vi "CRYRta weights interpolate.vi"(9 "Weights in dB":dbl[](array[numeric]) format="%.2f", 10 "Frequencies of weights array":dbl[](array[numeric]) format="%.2f", 11 "Nominal frequencies at this filter width":dbl[](array[numeric]) format="%.2f") -> (3 "dB-interpolated weights in linear squared":dbl[](array[numeric]) format="%.2f")   [LabVIEW 2013]
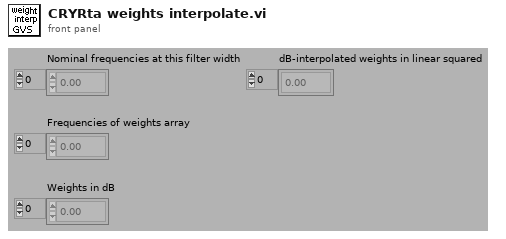
[diagram p1: front panel]
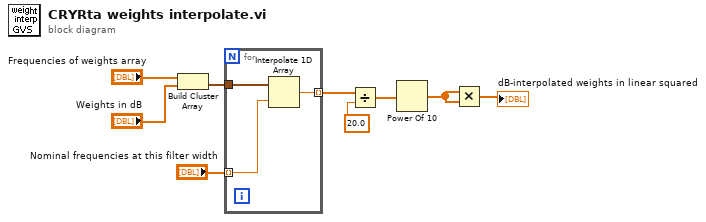
[diagram p0: block diagram]
diagram:
  n1 = Build Cluster Array("Frequencies of weights array", "Weights in dB") -> (w6:cluster{"Numeric":dbl, "Numeric":dbl}[])
  n2 = for {
    tunnel: "Nominal frequencies at this filter width" -> [w11] mode=indexing
    tunnel: w6 -> [w12]
    tunnel: [w10] -> w5 mode=indexing
    n3 = Interpolate 1D Array(1:w11, 2:w12) -> (0:w10:dbl)
  }
  n4 = Divide(x=w5, y=20.0) -> (x/y=w3:dbl[])
  n5 = Power Of 10(x=w3) -> (10^x=w2:dbl[])
  n6 = Multiply(x=w2, y=w2) -> (x*y=→"dB-interpolated weights in linear squared":dbl[])
